vi "Pedestrian Light Responsive.vi"() -> ()   [LabVIEW 2012]
doc: "Traffic Light VI with the use of Queues and LoadTrafficLightsQueue to Enqueue the Walk Element at the front of the initial State.\nNamed Second Loop as it uses second Loop to use an Event Structure with a Functional Global Boolean Variable to change the Waiting Indicator.\nTimeout Case has been implemented as with subVI that adds an Exit State to the end of the queue."
uses:
  Controls/Traffic Light Display.ctl
  Controls/Pedestrian Light Display.ctl
  Controls/Traffic Light States (with Walk and Exit State).ctl
  <vilib>/Utility/error.llb/DialogType.ctl
panel:
  out "Error String":string
  out "Waiting":bool
  in  "Stop Button":bool
  out "Pedestrian Light Display":T1
  in  "Walk":bool
  out "Traffic Light Display":T2
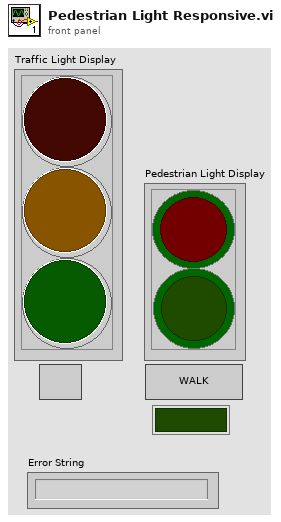
[diagram p1: front panel]
types:
  T1 = typedef "Pedestrian Light Display.ctl" = cluster{"Red":bool, "Green":bool}
  T2 = typedef "Traffic Light Display.ctl" = cluster{"RED":bool, "AMBER":bool, "GREEN":bool}
  T3 = typedef "Traffic Light States (with Walk and Exit State).ctl" = enum16{"Red", "RedAmber", "Green", "Amber", "Walk", "Exit"}
  T4 = typedef "DialogType.ctl" = u16
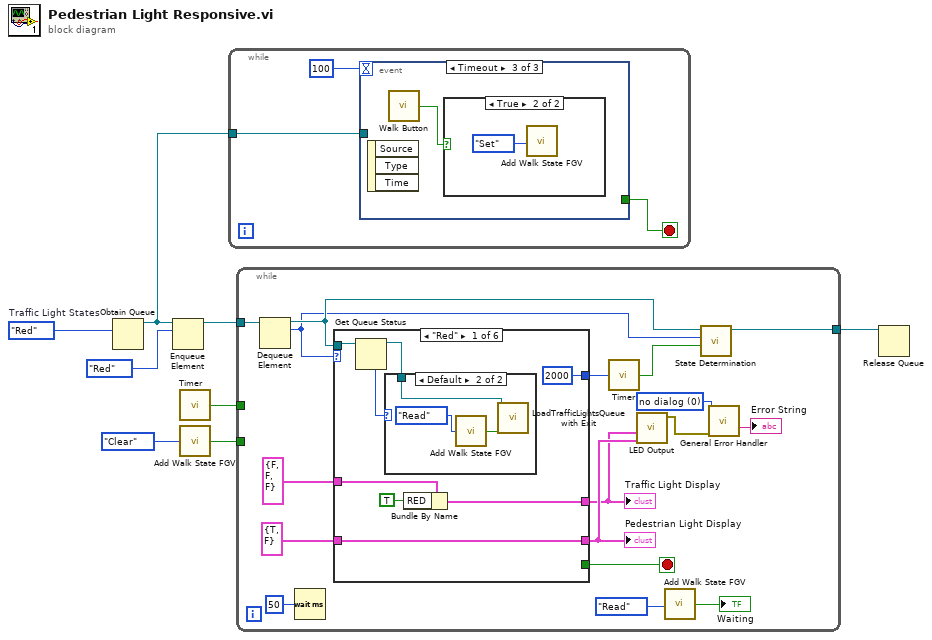
[diagram p0: block diagram]
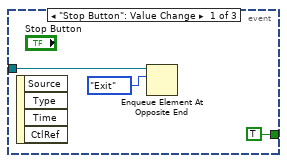
[diagram p2: hidden frame]
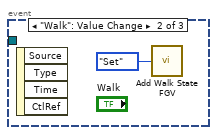
[diagram p3: hidden frame]
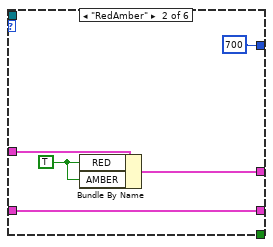
[diagram p6: hidden frame]
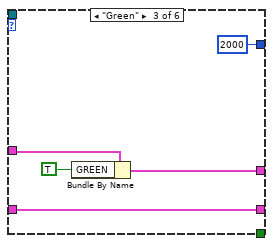
[diagram p7: hidden frame]
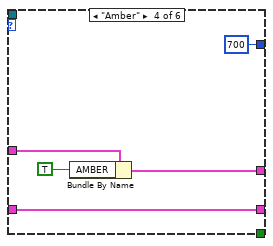
[diagram p8: hidden frame]
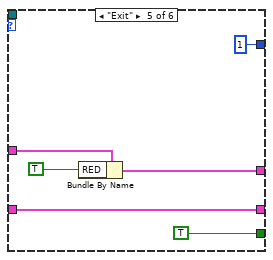
[diagram p9: hidden frame]
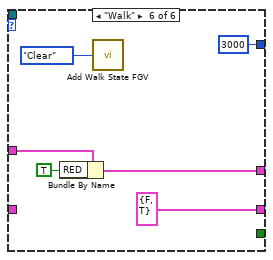
[diagram p10: hidden frame]
diagram:
  w6 = Traffic_Light_States_(with_Walk_and_Exit_State)."Red"  # Traffic Light States
  n1 = Obtain Queue(element data type=w6) -> (queue out=w7:refnum<queue>)  [unwired: 4 in, 2 out]
  n2 = Enqueue Element(queue=w7, element=Traffic_Light_States_(with_Walk_and_Exit_State)."Red" ("Traffic Light States")) -> (queue out=w8:refnum<queue>)  [unwired: 2 in, 2 out]
  n3 = call "Timer.vi"() -> ("Time Done"=w3:bool)  [unwired: 1 in]
  n4 = call "Add Walk State FGV.vi"("FGV Function"=enum16{"Clear", "Set", "Read"}."Clear") -> ("Boolean Indicator"=w1:bool)
  n5 = while {
    tunnel: w7 -> [w10]
    stop <- w11 stop-if-true
    n6 = event shown="[2] Timeout" {
      selector: _ -> [_ _ _]
      dyn-events: _ -> [_ _ _]
      timeout: 100 -> [_ _ _]
      tunnel: [TRUE _ _] -> w11
      tunnel: w10 -> [w13 _ _]
      event "Stop Button": Value Change {
        n7 = event-data() -> ()  [unwired: 1 in, 4 out]
        n8 = Enqueue Element At Opposite End(queue=w13, element=Traffic_Light_States_(with_Walk_and_Exit_State)."Exit" ("Traffic Light States")) -> ()  [unwired: 2 in, 3 out]
      }
      event "Walk": Value Change {
        n9 = event-data() -> ()  [unwired: 1 in, 4 out]
        n10 = call "Add Walk State FGV.vi"("FGV Function"=enum16{"Clear", "Set", "Read"}."Set") -> ()  [unwired: 1 out]
      }
      event Timeout {
        n11 = event-data() -> ()  [unwired: 1 in, 3 out]
        n12 = call "Walk Button.vi"() -> ("element"=w16:bool)  [unwired: 1 in]
        n13 = case shown="True" w16 {
          frame False {
          }
          frame True {
            n14 = call "Add Walk State FGV.vi"("FGV Function"=enum16{"Clear", "Set", "Read"}."Set") -> ()  [unwired: 1 out]
          }
        }
      }
    }
  }
  n15 = while {
    tunnel: w8 -> [w32]
    tunnel: [w26] -> w4
    tunnel: w3 -> [_]
    tunnel: w1 -> [_]
    stop <- w31 stop-if-true
    w18 = T4 0 items=["no dialog", "OK message", "continue or stop message", "OK message + warnings", "continue/stop + warnings"] ("type of dialog (OK msg:1)")
    n16 = Dequeue Element(queue=w32) -> (queue out=w28:refnum<queue>, element=w27:T3)  [unwired: 2 in, 2 out]
    n17 = Wait (ms)(milliseconds to wait=50) -> ()  [unwired: 1 out]
    n18 = case shown="\"Red\"" w27 {
      tunnel: T2 {"RED"=FALSE, "AMBER"=FALSE, "GREEN"=FALSE} ("Traffic Light Display") -> [w42 w50 w55 w60 w66 w71]
      tunnel: [w40 w49 w53 w58 w64 w69] -> w24
      tunnel: T1 {"Red"=TRUE, "Green"=FALSE} ("Pedestrian Light Display") -> [w39 w48 w52 w57 w63 _]
      tunnel: [w39 w48 w52 w57 w63 T1 {"Red"=FALSE, "Green"=TRUE} ("Pedestrian Light Display")] -> w25
      tunnel: w28 -> [w36 _ _ _ _ _]
      tunnel: [_ _ _ _ TRUE _] -> w31
      tunnel: [2000 700 2000 700 1 3000] -> w30
      frame "Red" {
        n19 = Get Queue Status(queue=w36) -> (queue out=w35:refnum<queue>, # elements in queue=w37:i32)  [unwired: 2 in, 6 out]
        n20 = case shown="Default" w37 {
          tunnel: w35 -> [_ w43]
          frame 5.. {
          }
          frame Default {
            n21 = call "Add Walk State FGV.vi"("FGV Function"=enum16{"Clear", "Set", "Read"}."Read") -> ("Boolean Indicator"=w44:bool)
            n22 = call "LoadTrafficLightsQueue with Exit.vi"("Queue Ref in"=w43, "Walk"=w44) -> ()  [unwired: 9 in]
          }
        }
        n23 = Bundle By Name(cluster=w42, "RED"=TRUE) -> (w40:T2)
      }
      frame "RedAmber" {
        w47 = TRUE ("RED")
        n24 = Bundle By Name(cluster=w50, "RED"=w47, "AMBER"=w47) -> (w49:T2)
      }
      frame "Green" {
        n25 = Bundle By Name(cluster=w55, "GREEN"=TRUE ("RED")) -> (w53:T2)
      }
      frame "Amber" {
        n26 = Bundle By Name(cluster=w60, "AMBER"=TRUE ("RED")) -> (w58:T2)
      }
      frame "Exit" {
        n27 = Bundle By Name(cluster=w66, "RED"=TRUE) -> (w64:T2)
      }
      frame "Walk" {
        n28 = Bundle By Name(cluster=w71, "RED"=TRUE) -> (w69:T2)
        n29 = call "Add Walk State FGV.vi"("FGV Function"=enum16{"Clear", "Set", "Read"}."Clear") -> ()  [unwired: 1 out]
      }
    }
    "Traffic Light Display" <- w24
    "Pedestrian Light Display" <- w25
    n30 = call "Timer.vi"("Wait Time (ms)"=w30) -> ("Time Done"=w29:bool)
    n31 = call "LED Output.vi"("Pedestrian Light Display"=w25, "Traffic Light Display"=w24) -> ("error out"=w19:errorcluster)  [unwired: 9 in]
    n32 = call "Add Walk State FGV.vi"("FGV Function"=enum16{"Clear", "Set", "Read"}."Read") -> ("Boolean Indicator"=→"Waiting":bool)
    n33 = call "State Determination.vi"("Time Done"=w29, "Current State"=w27, "Queue in"=w28) -> ("Queue out"=w26:refnum<queue>)  [unwired: 8 in]
    n34 = call <vilib>:"General Error Handler.vi"("type of dialog (OK msg:1)"=w18, "error in (no error)"=w19) -> ("message"=→"Error String":string)  [unwired: 9 in, 4 out]
  }
  n35 = Release Queue(queue=w4) -> ()  [unwired: 2 in, 3 out]
